vi "OCR_Set FG & BG Color first item in array.vi"(9 "Color Set":T1, 10 "Color Array":T1[](array[typedef])) -> (2 "Color Array":T1[](array[typedef]))   [LabVIEW 2009]
uses:
  Controls/Cluster/Cluster_Text Color Set.ctl
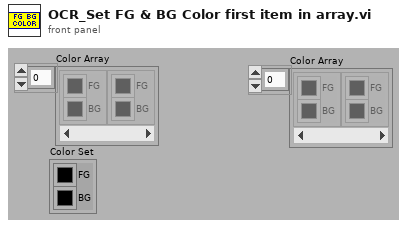
[diagram p1: front panel]
types:
  T1 = typedef "Cluster_Text Color Set.ctl" = cluster{"BG":u32, "FG":u32}
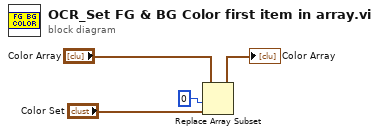
[diagram p0: block diagram]
diagram:
  n1 = Replace Array Subset(array="Color Array", new element="Color Set", index=0) -> (→"Color Array":T1[])
